vi "Notification.vi"(8 "error in (no error)":errorcluster, 11 "NotificationBarString":string="Test") -> (0 "error out":errorcluster)   [LabVIEW 2014]
uses:
  <vilib>/Utility/miscctls.llb/LVRectTypeDef.ctl
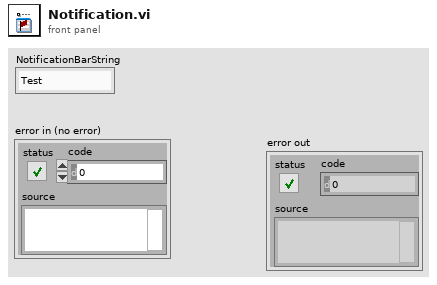
[diagram p1: front panel]
types:
  T1 = enum32{"Invalid", "Standard", "Closed", "Hidden", "Minimized", "Maximized"}
  T2 = typedef "LVRectTypeDef.ctl" = cluster{"Left":i16, "Top":i16, "Right":i16, "Bottom":i16}
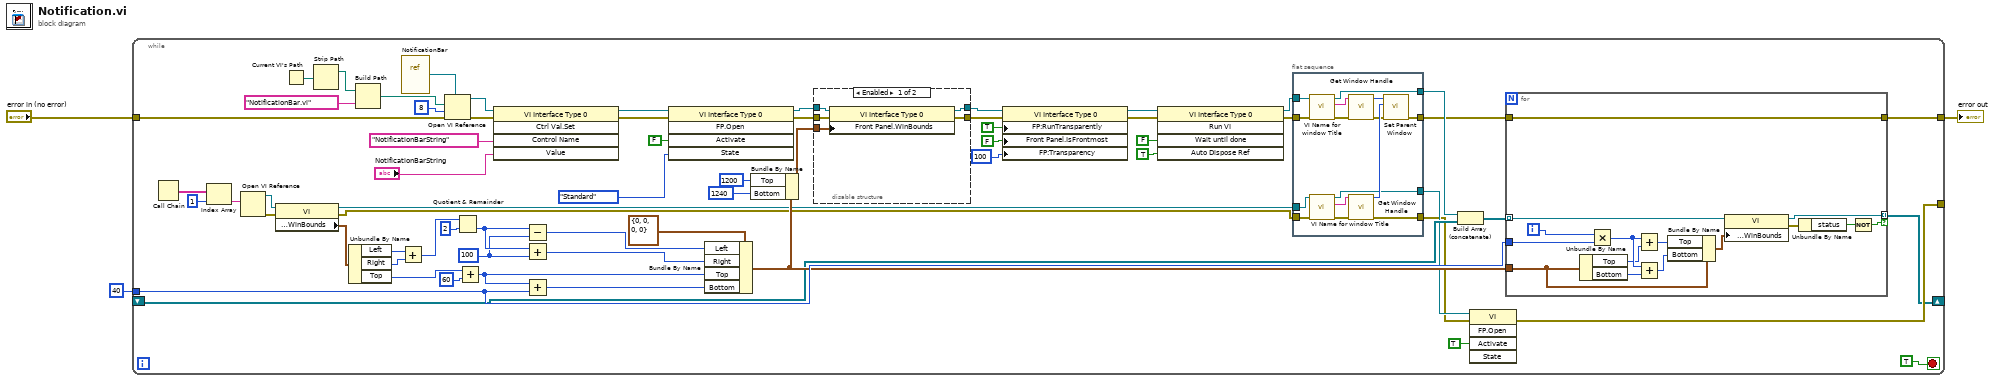
[diagram p0: block diagram]
diagram:
  n1 = while {
    shift-right: [w12] -> _
    shift-left: _ -> [w14]
    tunnel: "error in (no error)" -> [w58]
    tunnel: [w17] -> w2
    tunnel: i16 40 ("x") -> [w33]
    tunnel: [w16] -> _
    stop <- TRUE stop-if-true
    w41 = i16 100 ("y")
    n2 = Call Chain() -> (call chain=w68:string[])
    n3 = Index Array(array=w68, index=1) -> (element=w66:string)
    n4 = Open VI Reference(vi path=w66) -> (vi reference=w32:refnum<vi>, error out=w20:errorcluster)  [unwired: 5 in]
    n5 = property class="VI"(reference=w32, error in=w20) -> (reference out=w11:refnum<vi>, error out=w9:errorcluster, "Front Panel.WinBounds"=w47:T2)
    n6 = Current VI's Path() -> (path=w57:path)
    n7 = Strip Path(path=w57) -> (stripped path=w56:path)  [unwired: 1 out]
    n8 = Unbundle By Name(w47) -> ("Left"=w36:i16, "Right"=w37:i16, "Top"=w42:i16)
    n9 = Build Path(base path=w56, name or relative path="NotificationBar.vi") -> (appended path=w55:path)
    n10 = Add(x=w36, y=w37) -> (x+y=w38:i16)
    n11 = vi-ref "NotificationBar.vi"() -> (w65:refnum<vi>)
    n12 = Open VI Reference(type specifier VI Refnum (for type only)=w65, vi path=w55, options=8, error in (no error)=w58) -> (vi reference=w35:refnum<vi>, error out=w34:errorcluster)  [unwired: 2 in]
    n13 = Quotient & Remainder(x=w38, y=i16 2) -> (floor(x/y)=w44:i16)  [unwired: 1 out]
    n14 = Add(x=w42, y=i16 60) -> (x+y=w26:i16)
    n15 = invoke class="VI Interface Type 0" method="Ctrl Val.Set"(reference=w35, error in=w34, "Control Name"="NotificationBarString", "Value"="NotificationBarString") -> (reference out=w22:refnum<vi>, error out=w19:errorcluster)  [unwired: 1 in, 3 out]
    n16 = Subtract(x=w44, y=w41) -> (x-y=w28:i16)
    n17 = Add(x=w44, y=w41) -> (x+y=w27:i16)
    n18 = Add(x=w26, y=w33) -> (x+y=w25:i16)
    n19 = invoke class="VI Interface Type 0" method="FP.Open"(reference=w22, error in=w19, "Activate"=FALSE ("Activate?"), "State"=T1."Standard") -> (reference out=w50:refnum<vi>, error out=w52:errorcluster)  [unwired: 1 in, 3 out]
    n20 = Bundle By Name(cluster=T2 {"Left"=0, "Top"=0, "Right"=0, "Bottom"=0} ("Front Panel Window:Window Bounds"), "Left"=w28, "Right"=w27, "Top"=w26, "Bottom"=w25) -> (w24:T2)
    n21 = Bundle By Name(cluster=w24, "Top"=i16 1200, "Bottom"=i16 1240) -> (w7:T2)
    n22 = disable-structure shown="Enabled" {
      disable-tunnel: w52 -> [w73 _]
      disable-tunnel: w50 -> [w72 w74]
      disable-tunnel: [w71 _] -> w48
      disable-tunnel: [w70 w74] -> w46
      disable-tunnel: w7 -> [w69 _]
      frame Enabled {
        n23 = property class="VI Interface Type 0"(reference=w72, error in=w73, "Front Panel.WinBounds"=w69) -> (reference out=w70:refnum<vi>, error out=w71:errorcluster)
      }
      frame Disabled {
      }
    }
    n24 = property class="VI Interface Type 0"(reference=w46, error in=w48, "FP:RunTransparently"=TRUE ("Front Panel Window:Run VI Transparently"), "Front Panel.IsFrontmost"=FALSE ("Front Panel Window:Is Frontmost"), "FP:Transparency"=u8 100 ("Front Panel Window:Transparency")) -> (reference out=w21:refnum<vi>, error out=w15:errorcluster)
    n25 = invoke class="VI Interface Type 0" method="Run VI"(reference=w21, error in=w15, "Wait until done"=FALSE ("Wait Until Done"), "Auto Dispose Ref"=TRUE ("Auto Dispose Reference")) -> (reference out=w30:refnum<vi>, error out=w18:errorcluster)  [unwired: 1 in, 3 out]
    n26 = flat-sequence {
      tunnel: w11 -> [w84]
      tunnel: w30 -> [w83]
      tunnel: [w82] -> w29
      tunnel: [w81] -> w23
      tunnel: w18 -> [w80]
      tunnel: [w78] -> w10
      tunnel: w9 -> [w77]
      tunnel: [w75] -> w8
      frame #0 {
        n27 = call "VI Name for window Title.vi"("error in"=w80, "vi reference"=w83) -> ("error out"=w85:errorcluster, "Vi tiltle"=w88:string, "vi reference out (dup)"=w82:refnum<vi>)  [unwired: 7 out]
        n28 = call "VI Name for window Title.vi"("error in"=w77, "vi reference"=w84) -> ("error out"=w79:errorcluster, "Vi tiltle"=w89:string, "vi reference out (dup)"=w78:refnum<vi>)  [unwired: 7 out]
        n29 = call "Get Window Handle.vi"("error in (no error)"=w85, "window name (\"\")"=w88) -> ("error out"=w76:errorcluster, "hWnd"=w86:u32)  [unwired: 1 in, 3 out]
        n30 = call "Get Window Handle.vi"("error in (no error)"=w79, "window name (\"\")"=w89) -> ("error out"=w75:errorcluster, "hWnd"=w87:u32)  [unwired: 1 in, 3 out]
        n31 = call "Set Parent Window.vi"("error in (no error)"=w76, "new parent"=w87, "child"=w86) -> ("error out"=w81:errorcluster)  [unwired: 1 in, 7 out]
      }
    }
    n32 = Build Array (concatenate)(w29, w14) -> (w13:refnum<vi>[])
    n33 = invoke class="VI" method="FP.Open"(reference=w10, error in=w8, "Activate"=TRUE ("Activate?")) -> (error out=w16:errorcluster)  [unwired: 2 in, 4 out]
    n34 = for {
      tunnel: w13 -> [w95] mode=indexing
      tunnel: [w101] -> w12 mode=indexing if=w98
      tunnel: w33 -> [w97]
      tunnel: w24 -> [w94]
      tunnel: w23 -> [w91]
      tunnel: [w91] -> w17
      i -> [w90]
      n35 = Unbundle By Name(w94) -> ("Top"=w93:i16, "Bottom"=w92:i16)
      n36 = Multiply(x=w90, y=w97) -> (x*y=w96:i32)
      n37 = Add(x=w96, y=w93) -> (x+y=w103:i32)
      n38 = Add(x=w96, y=w92) -> (x+y=w102:i32)
      n39 = Bundle By Name(cluster=w94, "Top"=w103, "Bottom"=w102) -> (w104:T2)
      n40 = property class="VI"(reference=w95, "Front Panel.WinBounds"=w104) -> (reference out=w101:refnum<vi>, error out=w100:errorcluster)  [unwired: 1 in]
      n41 = Unbundle By Name(w100) -> ("status"=w99:bool)
      n42 = Not(x=w99) -> (.not. x?=w98:bool)
    }
  }
  "error out" <- w2
